vi "LastStepMsgParser.vi"(5 "Params array":string[](array[string]), 6 "Output Msg Table":string[][](table), 7 "Out MSG Codes":string[](array[string]), 8 "output msg array":cluster{i32, "Value":string, i32}[](array[cluster]), 9 "Out MSG Names":string[](array[string]), 10 "current msg num":i32) -> (2 "Params":string[](array[string]), 3 "code":i32[](array[numeric]), 4 "Output Alg Msg":string[][](table))   [LabVIEW 2009]
panel:
  out "Value":string
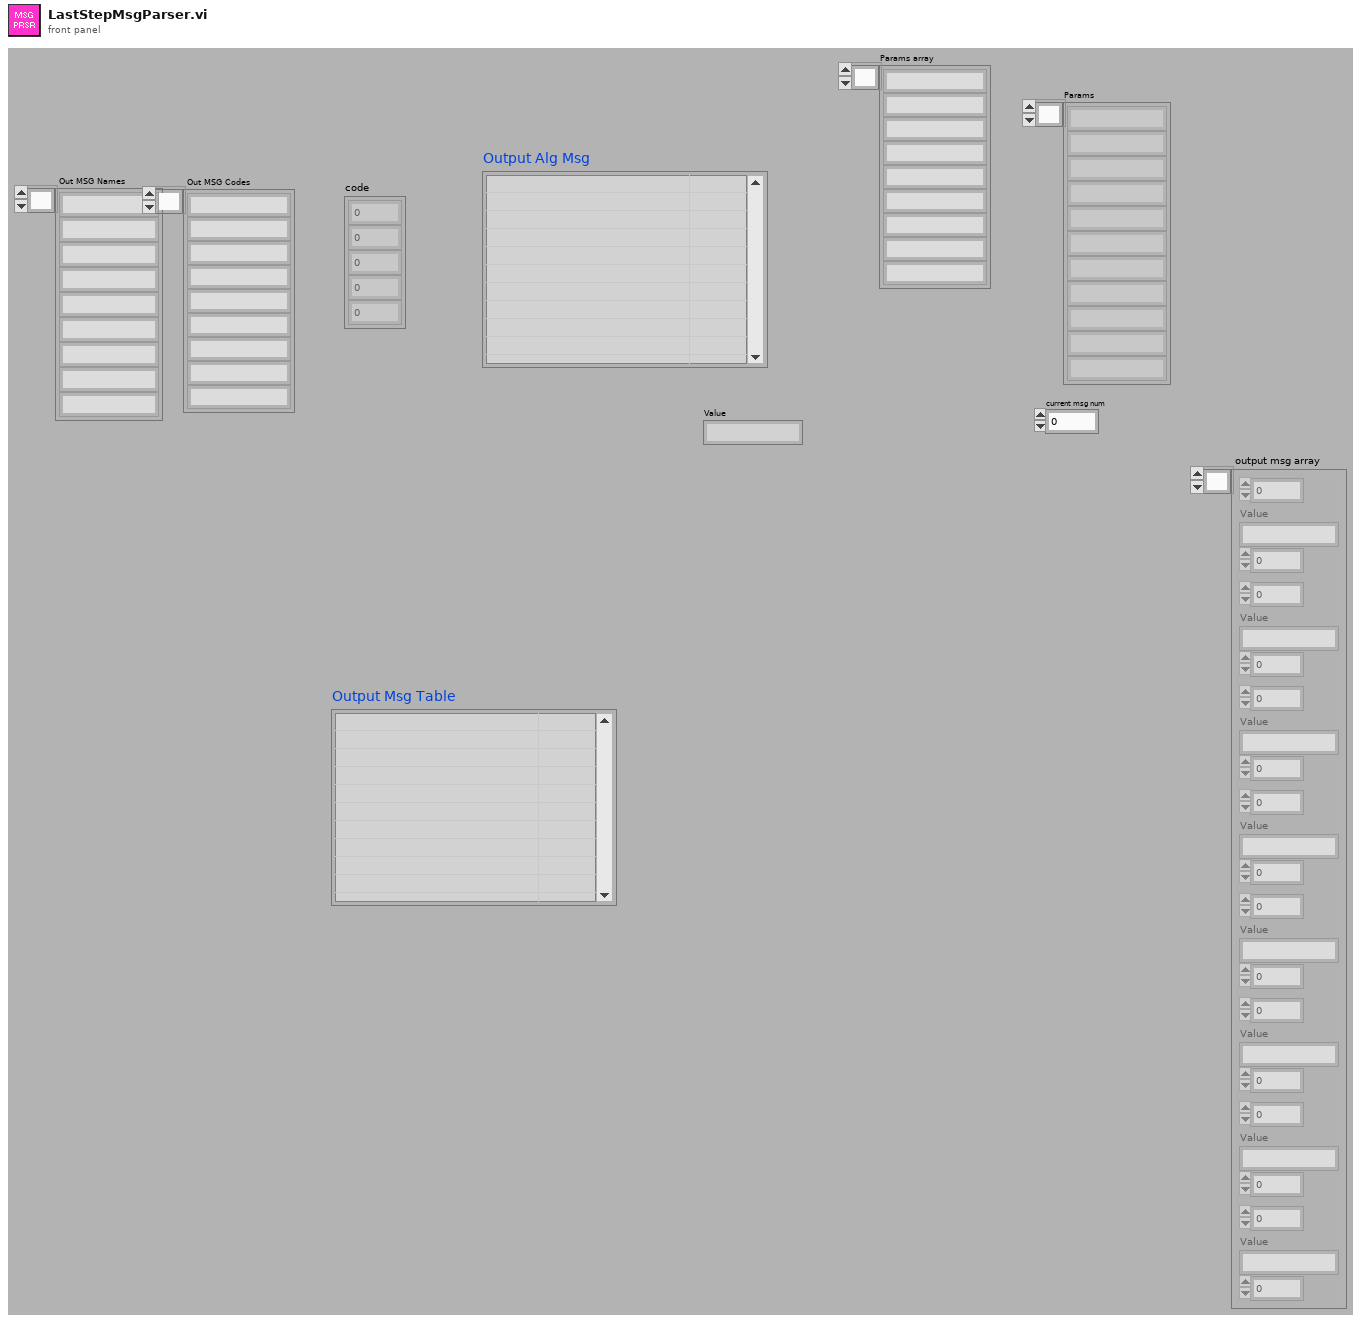
[diagram p1: front panel]
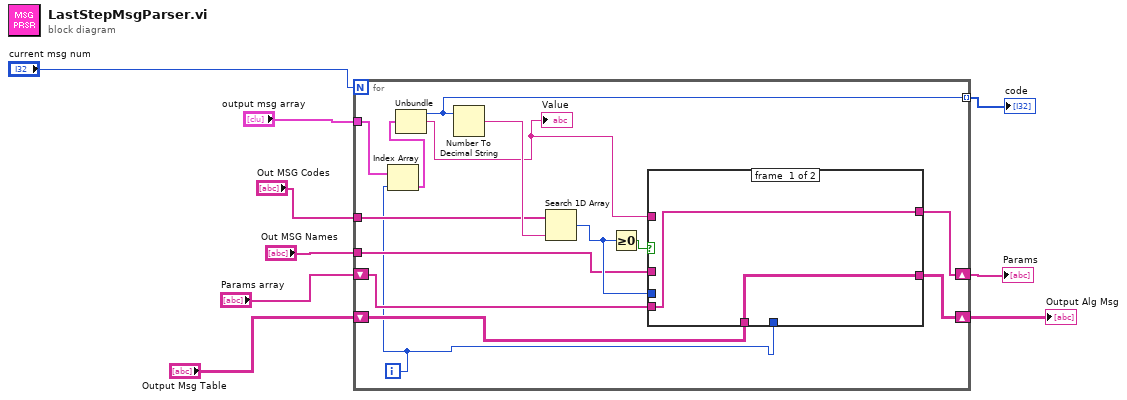
[diagram p0: block diagram]
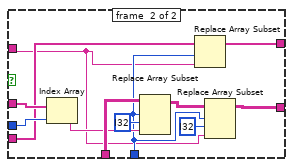
[diagram p2: hidden frame]
diagram:
  n1 = for {
    N: "current msg num" -> [_]
    tunnel: "output msg array" -> [w14]
    tunnel: [w23] -> w7 mode=indexing
    shift-right: [w18] -> w1
    shift-left: "Output Msg Table" -> [w19]
    tunnel: "Out MSG Codes" -> [w17]
    tunnel: "Out MSG Names" -> [w16]
    shift-right: [w11] -> w3
    shift-left: "Params array" -> [w12]
    i -> [w10]
    n2 = Index Array(array=w14, index=w10) -> (element=w13:cluster{i32, "Value":string, i32})
    n3 = Unbundle(w13) -> (w23:i32, "Value"=w15:string)  [unwired: 1 out]
    "Value" <- w15
    n4 = Number To Decimal String(number=w23) -> (decimal integer string=w22:string)  [unwired: 1 in]
    n5 = Search 1D Array(1D array=w17, element=w22) -> (index of element=w20:i32)  [unwired: 1 in]
    n6 = Greater Or Equal To 0?(x=w20) -> (x >= 0?=w21:bool)
    n7 = case shown="True" w21 {
      tunnel: w16 -> [_ w37]
      tunnel: w20 -> [_ w36]
      tunnel: w15 -> [_ w27]
      tunnel: w19 -> [w25 w35]
      tunnel: [w25 w31] -> w18
      tunnel: w10 -> [_ w28]
      tunnel: w12 -> [w24 w29]
      tunnel: [w24 w26] -> w11
      frame #0 {
      }
      frame #1 {
        n8 = Index Array(array=w37, index=w36) -> (element=w34:string)
        n9 = Replace Array Subset(array=w35, new element=w34, index (row)=w28, index (col)=i32 ? ("disabled index (col)")) -> (w30:string[][])
        n10 = Replace Array Subset(array=w29, new element=w27, index=w28) -> (w26:string[])
        n11 = Replace Array Subset(array=w30, new element=w27, index (row)=w28, index (col)=i32 ? ("disabled index (col)")) -> (w31:string[][])
      }
    }
  }
  "code" <- w7
  "Output Alg Msg" <- w1
  "Params" <- w3
